vi "DriveForward.vi"(0 "LeftEncoder":T11={"DevStatus"={"status"=FALSE, "code"=0, "source"=""}, "EncoderIndex"=enum."Invalid", "CounterIndex"=enum."Invalid", "DistancePerCount"=1.0, "Decoding Type"=enum."4x"}, 1 "RightEncoder":T11={"DevStatus"={"status"=FALSE, "code"=0, "source"=""}, "EncoderIndex"=enum."Invalid", "CounterIndex"=enum."Invalid", "DistancePerCount"=1.0, "Decoding Type"=enum."4x"}, 2 "Inches to Travel":dbl, 3 "BackDrive":T1={"DevStatus"={"status"=FALSE, "code"=0, "source"=""}, "Motors[]"=[], "Square Inputs"=FALSE, "Max Output"=1.0}, 4 "FrontDrive":T1={"DevStatus"={"status"=FALSE, "code"=0, "source"=""}, "Motors[]"=[], "Square Inputs"=FALSE, "Max Output"=1.0}, 5 "error in":errorcluster) -> (6 "error out":errorcluster)   [LabVIEW 2014]
uses:
  <vilib>/Rock Robotics/WPI/RobotDrive/WPI_RobotDriveDevRef.ctl
  <vilib>/Rock Robotics/WPI/MotorControl/WPI_MotorControlDeviceRef.ctl
  <vilib>/Rock Robotics/WPI/MotorControl/WPI_MotorControlType.ctl
  <vilib>/Rock Robotics/SystemInterfaces/Typedef/FPGA_TypedefDigitalModule.ctl
  <vilib>/Rock Robotics/SystemInterfaces/DIO/FPGA_DIOPWMChannel.ctl
  <vilib>/Rock Robotics/WPI/PWM/WPI_PWMDeadband.ctl
  <vilib>/Rock Robotics/WPI/CAN/Jaguar/SubVIs/WPI_CANJaguar_ControlMode.ctl
  <vilib>/Rock Robotics/WPI/CAN/TalonSRX/WPI_CANTalonSRX_APIControlMode.ctl
  <vilib>/Rock Robotics/WPI/PWM/WPI_PWMTransform_ConPane.ctl
  <vilib>/Rock Robotics/WPI/Encoder/WPI_EncoderDevRef.ctl
  <vilib>/Rock Robotics/SystemInterfaces/Encoder/FPGA_EncoderIdx.ctl
  <vilib>/Rock Robotics/SystemInterfaces/Counter/FPGA_CounterCtrSystemIndex.ctl
  <vilib>/Rock Robotics/WPI/Encoder/WPI_EncoderType.ctl
  <vilib>/addons/control/pid/pid.llb/PID (DBL).vi
  <vilib>/addons/control/pid/NI_PID_pid.lvlib
panel:
  out "x-y":dbl
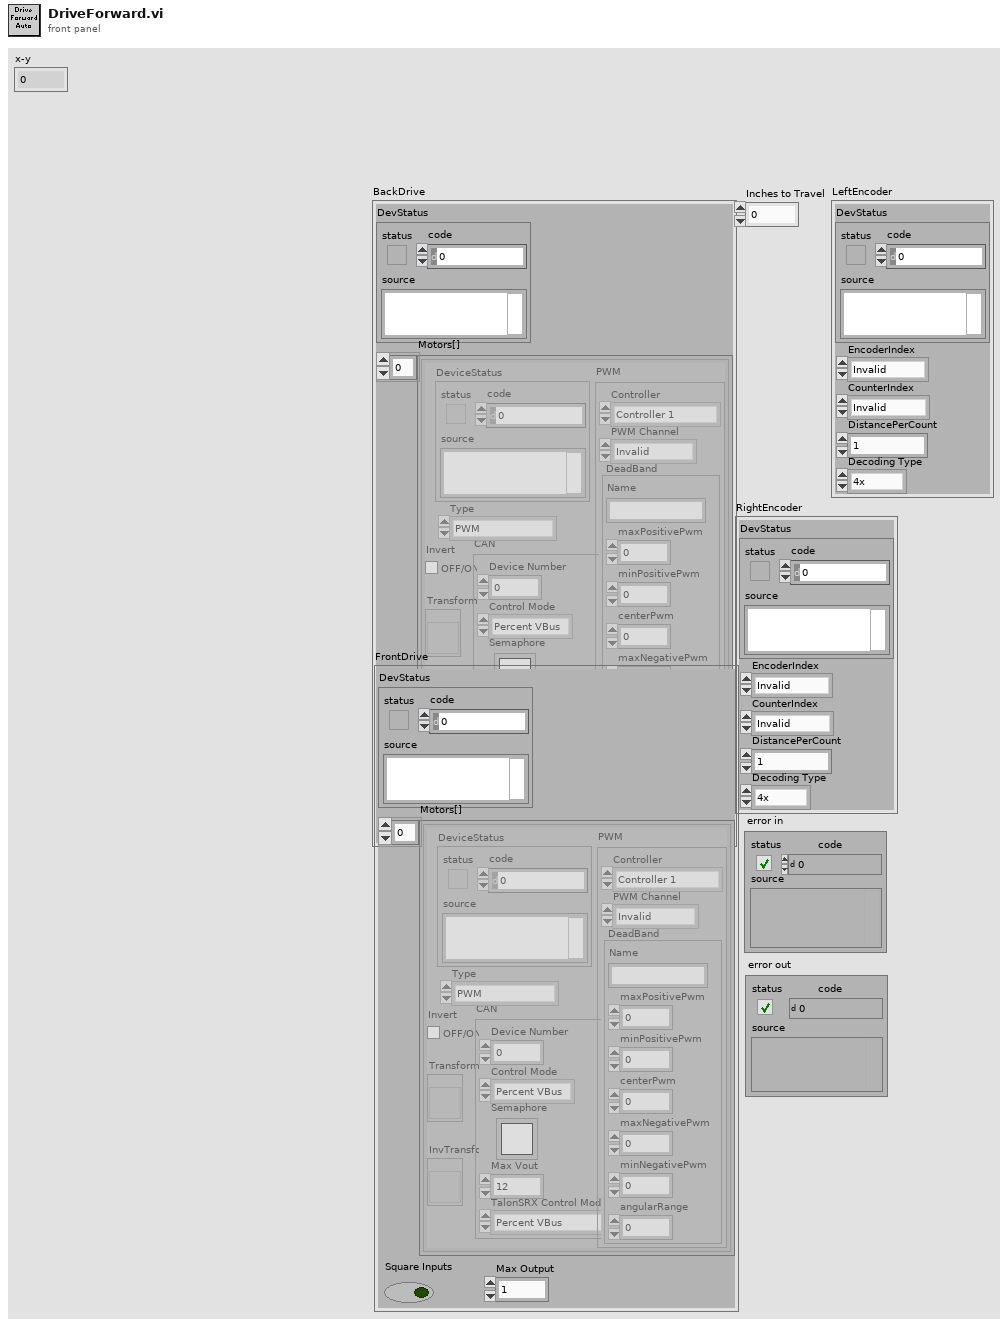
[diagram p1: front panel]
types:
  T1 = typedef "WPI_RobotDriveDevRef.ctl" = cluster{"DevStatus":errorcluster, "Motors[]":T2[], "Square Inputs":bool, "Max Output":dbl}
  T2 = typedef "WPI_MotorControlDeviceRef.ctl" = cluster{"DeviceStatus":errorcluster, "Type":T3, "PWM":cluster{"Controller":T4, "PWM Channel":T5, "DeadBand":T6}, "CAN":cluster{"Device Number":u8, "Control Mode":T7, "Semaphore":T8, "Max Vout":dbl, "TalonSRX Control Mode":T9}, "Invert":bool, "TransformRef":T10, "InvTransformRef":T10}
  T3 = typedef "WPI_MotorControlType.ctl" = enum16{"PWM", "CAN", "CANTalonSRX"}
  T4 = typedef "FPGA_TypedefDigitalModule.ctl" = enum16{"Controller 1"}
  T5 = typedef "FPGA_DIOPWMChannel.ctl" = enum8{"PWM 0", "PWM 1", "PWM 2", "PWM 3", "PWM 4", "PWM 5", "PWM 6", "PWM 7", "PWM 8", "PWM 9", "PWM MXP 0", "PWM MXP 1", "PWM MXP 2", "PWM MXP 3", "PWM MXP 4", "PWM MXP 5", "PWM MXP 6", "PWM MXP 7", "PWM MXP 8", "PWM MXP 9", "Invalid"}
  T6 = typedef "WPI_PWMDeadband.ctl" = cluster{"Name":string, "maxPositivePwm":i32, "minPositivePwm":i32, "centerPwm":i32, "maxNegativePwm":i32, "minNegativePwm":i32, "angularRange":u16}
  T7 = typedef "WPI_CANJaguar_ControlMode.ctl" = enum8{"Percent VBus", "Current", "Speed", "Position", "Voltage"}
  T8 = typedef "Semaphore RefNum" = refnum<k1>
  T9 = typedef "WPI_CANTalonSRX_APIControlMode.ctl" = enum8{"Percent VBus", "Speed", "Position", "Slave", "Unchanged / Invalid"}
  T10 = typedef "WPI_PWMTransform_ConPane.ctl" = refnum<vi>
  T11 = typedef "WPI_EncoderDevRef.ctl" = cluster{"DevStatus":errorcluster, "EncoderIndex":T12, "CounterIndex":T13, "DistancePerCount":dbl, "Decoding Type":T14}
  T12 = typedef "FPGA_EncoderIdx.ctl" = enum8{"Enc 0", "Enc 1", "Enc 2", "Enc 3", "Enc 4", "Enc 5", "Enc 6", "Enc 7", "Invalid"}
  T13 = typedef "FPGA_CounterCtrSystemIndex.ctl" = enum8{"Ctr 0", "Ctr 1", "Ctr 2", "Ctr 3", "Ctr 4", "Ctr 5", "Ctr 6", "Ctr 7", "Invalid"}
  T14 = typedef "WPI_EncoderType.ctl" = enum16{"1x", "2x", "4x"}
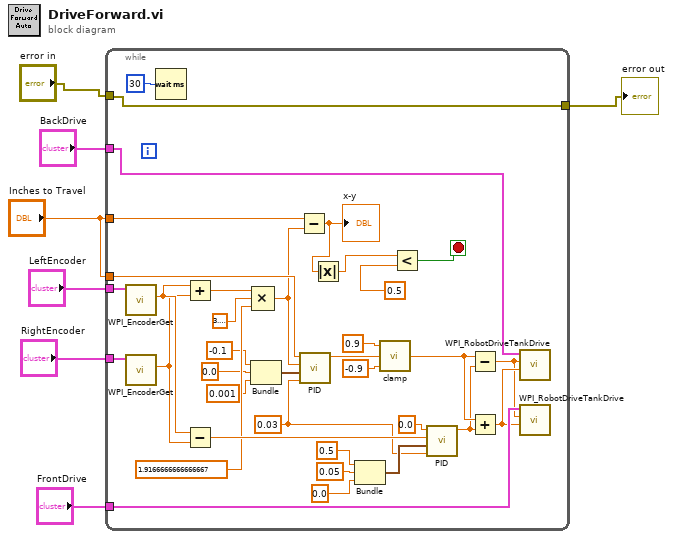
[diagram p0: block diagram]
diagram:
  n1 = while {
    tunnel: "Inches to Travel" -> [w28]
    tunnel: "LeftEncoder" -> [w27]
    tunnel: "RightEncoder" -> [w26]
    tunnel: "FrontDrive" -> [w22]
    tunnel: "BackDrive" -> [w21]
    tunnel: "Inches to Travel" -> [w9]
    tunnel: "error in" -> [w8]
    tunnel: [w8] -> w1
    stop <- w10 stop-if-true
    w23 = 0.03 ("dt (s)")
    n2 = call <vilib>:"WPI_EncoderGet.vi"("EncoderDevRef"=w27) -> ("Distance"=w37:dbl)  [unwired: 5 in, 5 out]
    n3 = call <vilib>:"WPI_EncoderGet.vi"("EncoderDevRef"=w26) -> ("Distance"=w36:dbl)  [unwired: 5 in, 5 out]
    n4 = Wait (ms)(milliseconds to wait=u32 30) -> ()  [unwired: 1 out]
    n5 = Add(x=w37, y=w36) -> (x+y=w35:dbl)
    n6 = Subtract(x=w37, y=w36) -> (x-y=w38:dbl)
    n7 = Bundle(-0.1, 0.0, 0.001) -> (w30:cluster{dbl, dbl, dbl})  [unwired: 1 in]
    n8 = Compound Arithmetic op=MULTIPLY(w35, 3.141592653589793, 1.9166666666666667 ("value")) -> (w20:dbl)
    n9 = Subtract(x=w9, y=w20) -> (x-y=w11:dbl)
    "x-y" <- w11
    n10 = call-poly <vilib>:"PID.vi"("dt (s)"=w23, "PID gains"=w30, "process variable"=w20, "setpoint"=w28) -> ("output"=w18:dbl)  [unwired: 6 in, 1 out]
    n11 = Absolute Value(x=w11) -> (abs(x)=w12:dbl)
    n12 = Bundle(0.5, 0.05, 0.0) -> (w40:cluster{dbl, dbl, dbl})  [unwired: 1 in]
    n13 = call "clamp.vi"("Min"=-0.9, "Input"=w18, "Max"=0.9) -> ("Output"=w17:dbl)
    n14 = Less?(x=w12, y=0.5) -> (x < y?=w10:bool)
    n15 = call-poly <vilib>:"PID.vi"("dt (s)"=w23, "PID gains"=w40, "process variable"=w38, "setpoint"=0.0) -> ("output"=w16:dbl)  [unwired: 6 in, 1 out]
    n16 = Subtract(x=w17, y=w16) -> (x-y=w14:dbl)
    n17 = Add(x=w17, y=w16) -> (x+y=w15:dbl)
    n18 = call <vilib>:"WPI_RobotDriveTankDrive.vi"("Right axis value"=w15, "Left axis value"=w14, "RobotDriveDevRef"=w21) -> ()  [unwired: 6 in, 3 out]
    n19 = call <vilib>:"WPI_RobotDriveTankDrive.vi"("Right axis value"=w15, "Left axis value"=w14, "RobotDriveDevRef"=w22) -> ()  [unwired: 6 in, 3 out]
  }
  "error out" <- w1
